vi "S8300E_BOOTUP_ChkKeyWord_new.vi"() -> ()   [LabVIEW 2011]
panel:
  out "Found S8300e login":bool
  out "start check time":u32
  out "Time Elpased (sec 秒)":dbl
  out "Found  keyword?":bool
  out "Debug View":string
  out "VISA resource name out":refnum<visa-resource-name>
  out "進行狀況":string
  out "BEGIN TIME":u32
  # "Error Code:USB-IF1"
  # "S8300E Check keyword"
  # "2015-3-5"
  # "COM9 115200"
  # "1.本程式不會給UUT 上電,需先執行上電程式\n2.本程式只檢查特定字串後按迴車鍵"
  # "開機穩定需花2分鐘\nWait for 2 mins for system ready"
  # "Write Command :Char by Char"
  # "一律由U盤開機"
  # "Deallocates unused memory \nafter the SW program exit"
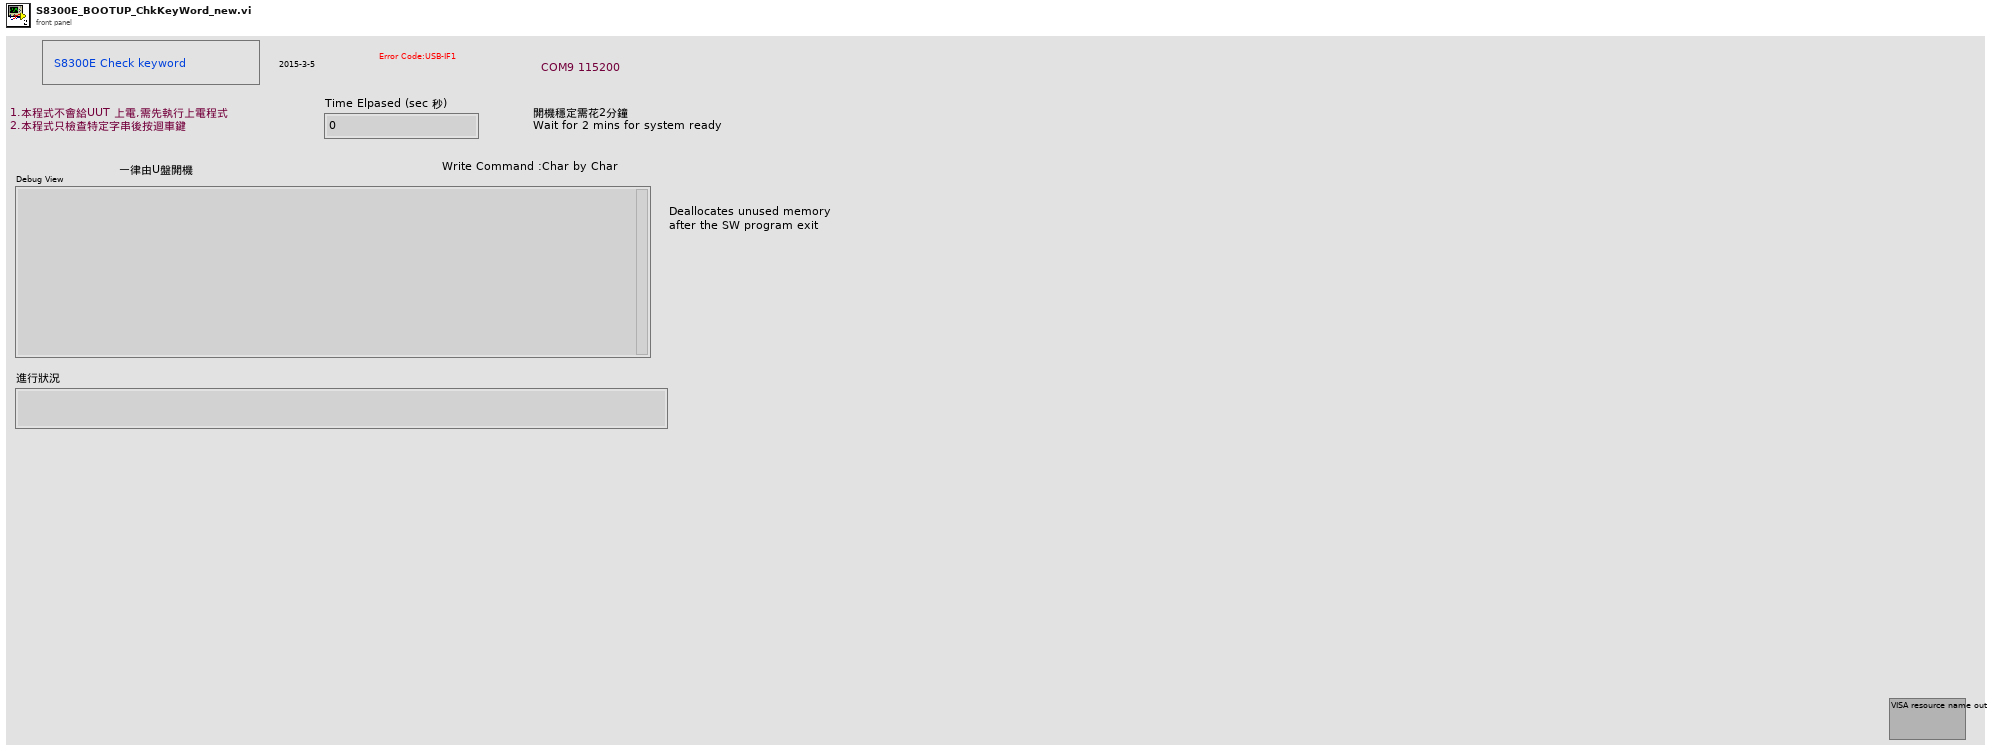
[diagram p1: front panel]
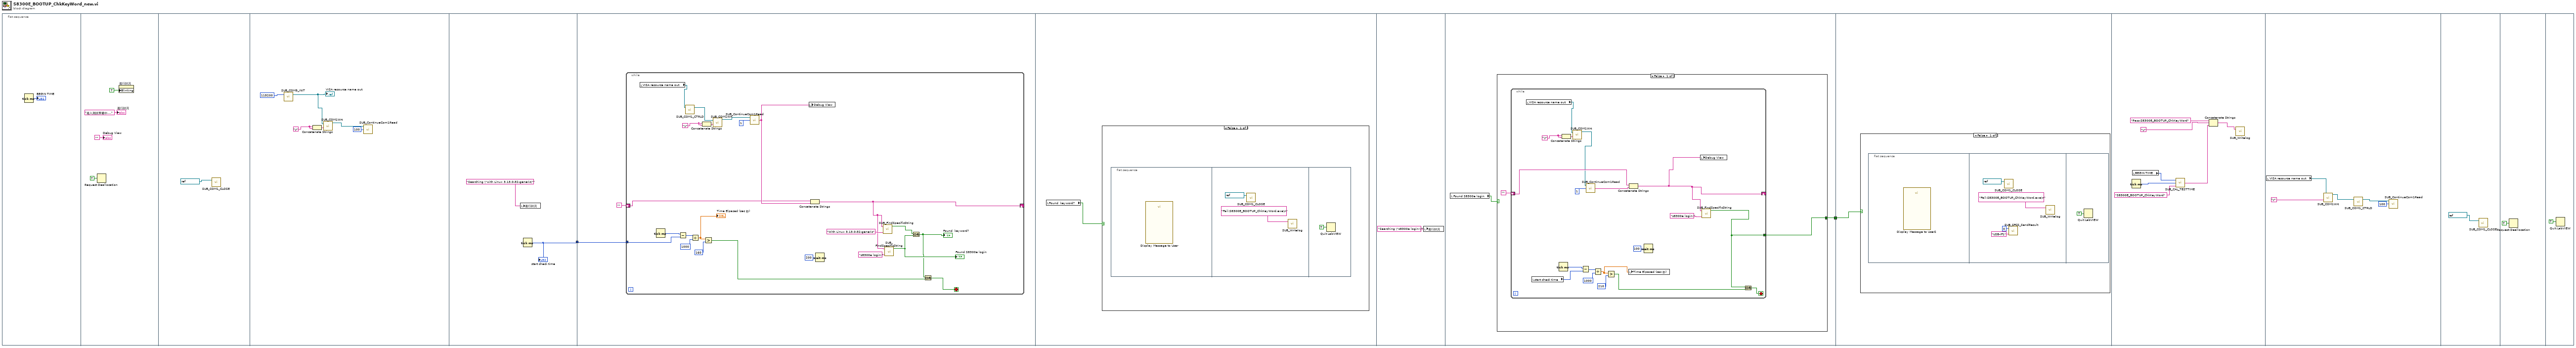
[diagram p0: block diagram]
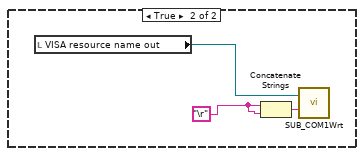
[diagram p2: hidden frame]
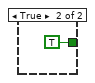
[diagram p3: hidden frame]
diagram:
  n1 = flat-sequence {
    tunnel: [w16] -> w2
    tunnel: w2 -> [w18]
    tunnel: [w51] -> w1
    tunnel: w1 -> [w74]
    frame #0 {
      n2 = Tick Count (ms)() -> (millisecond timer value=→"BEGIN TIME":u32)
    }
    frame #1 {
      n3 = Request Deallocation(TRUE ("flag")) -> ()
      n4 = property on="進行狀況" class="Str"("Blinking"=TRUE) -> ()  [unwired: 2 in, 2 out]
      "進行狀況" <- "進入測試準備中...." ("進行狀況")
      "Debug View" <- ""
    }
    frame #2 {
      n5 = call "SUB_COM1_CLOSE.vi"("VISA resource name"=refnum<visa-resource-name> "COM9") -> ()  [unwired: 3 in]
    }
    frame #3 {
      w11 = "\r"
      n6 = call "SUB_COM9_INIT.vi"("baud rate"=u32 115200) -> ("VISA resource name out"=w13:refnum<visa-resource-name>)  [unwired: 1 in, 1 out]
      "VISA resource name out" <- w13
      n7 = Concatenate Strings(w11, w11) -> (w12:string)
      n8 = call "SUB_COM1Wrt.vi"("VISA resource name"=w13, "write buffer"=w12) -> ("duplicate VISA resource name"=w10:refnum<visa-resource-name>)  [unwired: 1 in, 1 out]
      n9 = call "SUB_ContinueCom1Read.vi"("Numeric"=100, "duplicate VISA resource name 2"=w10) -> ()  [unwired: 1 in, 3 out]
    }
    frame #4 {
      n10 = local write "進行狀況"("Searching \"with Linux 3.13.0-32-generic\"" ("進行狀況")) -> ()
      n11 = Tick Count (ms)() -> (millisecond timer value=w16:u32)
      "start check time" <- w16
    }
    frame #5 {
      n12 = while {
        shift-right: [w26] -> _
        shift-left: "" -> [w39]
        tunnel: w18 -> [w37]
        stop <- w31 stop-if-true
        w28 = "\r"
        n13 = local read "VISA resource name out"() -> (w21:refnum<visa-resource-name>)
        n14 = Tick Count (ms)() -> (millisecond timer value=w38:u32)
        n15 = Subtract(x=w38, y=w37) -> (x-y=w36:u32)
        n16 = call "SUB_COM1_CTRLD.vi"("VISA resource name"=w21) -> ("duplicate VISA resource name"=w20:refnum<visa-resource-name>)  [unwired: 1 in, 1 out]
        n17 = Divide(x=w36, y=u32 1000) -> (x/y=w34:dbl)
        "Time Elpased (sec 秒)" <- w34
        n18 = Concatenate Strings(w28, w28) -> (w29:string)
        n19 = Greater?(x=w34, y=u32 160) -> (0:w32:bool)
        n20 = call "SUB_COM1Wrt.vi"("VISA resource name"=w20, "write buffer"=w29) -> ("duplicate VISA resource name"=w27:refnum<visa-resource-name>)  [unwired: 1 in, 1 out]
        n21 = call "SUB_ContinueCom1Read.vi"("Numeric"=1, "duplicate VISA resource name 2"=w27) -> ("String"=w40:string)  [unwired: 1 in, 2 out]
        n22 = local write "Debug View"(w40) -> ()
        n23 = Concatenate Strings(w39, w40) -> (w26:string)
        n24 = Wait (ms)(milliseconds to wait=u32 200) -> ()  [unwired: 1 out]
        n25 = call "SUB_FindSpecificString.vi"("Find this String"="With Linux 3.13.0-32-generic", "String data"=w26) -> ("Found"=w24:bool)  [unwired: 2 in, 1 out]
        n26 = call "SUB_FindSpecificString.vi"("Find this String"="s8300e login:", "String data"=w26) -> ("Found"=w23:bool)  [unwired: 2 in, 1 out]
        "Found S8300e login" <- w23
        n27 = Or(x=w24, y=w23) -> (x .or. y?=w22:bool)
        "Found  keyword?" <- w22
        n28 = Or(x=w22, y=w32) -> (x .or. y?=w31:bool)
      }
    }
    frame #6 {
      n29 = local read "Found  keyword?"() -> (w42:bool)
      n30 = case shown="False" w42 {
        frame False {
          n31 = flat-sequence {
            frame #0 {
              n32 = call "Display Message to User"() -> ()  [unwired: 10 in, 2 out]
            }
            frame #1 {
              n33 = call "SUB_COM1_CLOSE.vi"("VISA resource name"=refnum<visa-resource-name> "COM9") -> ()  [unwired: 3 in]
              n34 = call "SUB_Writelog.vi"("Pass/Fail"="Fail:S8300E_BOOTUP_ChkKeyWord.exe\n") -> ()  [unwired: 2 in]
            }
            frame #2 {
              n35 = Quit LabVIEW(quit? (T)=TRUE) -> ()
            }
          }
        }
        frame True {
          w47 = "\r"
          n36 = local read "VISA resource name out"() -> (w48:refnum<visa-resource-name>)
          n37 = Concatenate Strings(w47, w47) -> (w46:string)
          n38 = call "SUB_COM1Wrt.vi"("VISA resource name"=w48, "write buffer"=w46) -> ()  [unwired: 1 in, 2 out]
        }
      }
    }
    frame #7 {
      n39 = local write "進行狀況"("Searching \"s8300e login:\"" ("進行狀況")) -> ()
    }
    frame #8 {
      n40 = local read "Found S8300e login"() -> (w50:bool)
      n41 = case shown="False" w50 {
        tunnel: [w52 TRUE ("Found")] -> w51
        frame False {
          n42 = while {
            shift-right: [w60] -> _
            shift-left: "" -> [w65]
            tunnel: [w59] -> w52
            stop <- w62 stop-if-true
            w57 = "\r"
            n43 = local read "VISA resource name out"() -> (w56:refnum<visa-resource-name>)
            n44 = local read "start check time"() -> (w63:u32)
            n45 = Tick Count (ms)() -> (millisecond timer value=w68:u32)
            n46 = Concatenate Strings(w57, w57) -> (w58:string)
            n47 = call "SUB_COM1Wrt.vi"("VISA resource name"=w56, "write buffer"=w58) -> ("duplicate VISA resource name"=w55:refnum<visa-resource-name>)  [unwired: 1 in, 1 out]
            n48 = Subtract(x=w68, y=w63) -> (x-y=w69:u32)
            n49 = call "SUB_ContinueCom1Read.vi"("Numeric"=1, "duplicate VISA resource name 2"=w55) -> ("String"=w66:string)  [unwired: 1 in, 2 out]
            n50 = Divide(x=w69, y=u32 1000) -> (x/y=w64:dbl)
            n51 = Greater?(x=w64, y=u32 210) -> (0:w61:bool)
            n52 = local write "Time Elpased (sec 秒)"(w64) -> ()
            n53 = Concatenate Strings(w65, w66) -> (w60:string)
            n54 = Wait (ms)(milliseconds to wait=u32 100) -> ()  [unwired: 1 out]
            n55 = local write "Debug View"(w60) -> ()
            n56 = call "SUB_FindSpecificString.vi"("Find this String"="s8300e login:", "String data"=w60) -> ("Found"=w59:bool)  [unwired: 2 in, 1 out]
            n57 = Or(x=w59, y=w61) -> (x .or. y?=w62:bool)
          }
        }
        frame True {
        }
      }
    }
    frame #9 {
      n58 = case shown="False" w74 {
        frame False {
          n59 = flat-sequence {
            frame #0 {
              n60 = call "Display Message to User2"() -> ()  [unwired: 10 in, 2 out]
            }
            frame #1 {
              n61 = call "SUB_COM1_CLOSE.vi"("VISA resource name"=refnum<visa-resource-name> "COM9") -> ()  [unwired: 3 in]
              n62 = call "SUB_SFCS_SendResult.vi"("ErrorCode"="USB-IF1", "PASS_Fail (1/0)"=i8 0) -> ()  [unwired: 1 out]
              n63 = call "SUB_Writelog.vi"("Pass/Fail"="Fail:S8300E_BOOTUP_ChkKeyWord.exe\n") -> ()  [unwired: 2 in]
            }
            frame #2 {
              n64 = Quit LabVIEW(quit? (T)=TRUE) -> ()
            }
          }
        }
        frame True {
        }
      }
    }
    frame #10 {
      n65 = Tick Count (ms)() -> (millisecond timer value=w84:u32)
      n66 = local read "BEGIN TIME"() -> (w85:u32)
      n67 = call "SUB_CAL_TESTTIME.vi"("Test Item name"="S8300E_BOOTUP_ChkKeyWord", "Stop tick time"=w84, "Start tick time"=w85) -> ("Test Time output"=w80:string)  [unwired: 2 in]
      n68 = Concatenate Strings("Pass:S8300E_BOOTUP_ChkKeyWord" ("string"), "\r", w80) -> (w82:string)
      n69 = call "SUB_Writelog.vi"("Pass/Fail"=w82) -> ()  [unwired: 2 in]
    }
    frame #11 {
      n70 = local read "VISA resource name out"() -> (w89:refnum<visa-resource-name>)
      n71 = call "SUB_COM1Wrt.vi"("VISA resource name"=w89, "write buffer"="\r") -> ("duplicate VISA resource name"=w91:refnum<visa-resource-name>)  [unwired: 1 in, 1 out]
      n72 = call "SUB_COM1_CTRLD.vi"("VISA resource name"=w91) -> ("duplicate VISA resource name"=w88:refnum<visa-resource-name>)  [unwired: 1 in, 1 out]
      n73 = call "SUB_ContinueCom1Read.vi"("Numeric"=100, "duplicate VISA resource name 2"=w88) -> ()  [unwired: 1 in, 3 out]
    }
    frame #12 {
      n74 = call "SUB_COM1_CLOSE.vi"("VISA resource name"=refnum<visa-resource-name> "COM9") -> ()  [unwired: 3 in]
    }
    frame #13 {
      n75 = Request Deallocation(TRUE ("flag")) -> ()
    }
    frame #14 {
      n76 = Quit LabVIEW(quit? (T)=TRUE) -> ()
    }
  }
